vi "ReadAI.vi"(8 "error in (no error)":errorcluster, 11 "FPGA VI Reference In":refnum<k20>) -> (0 "error out":errorcluster, 2 "AI_readValues":dbl[](array[numeric]), 3 "FPGA VI Reference Out":refnum<k20>)   [LabVIEW 2020, in "FPGA_IO.lvlib"]
doc: "Read AI values from the FPGA\nChannels: C/AI0, C/AI1"
uses:
  FPGA_IO.lvlib
  <vilib>/Utility/error.llb/Error Cluster From Error Code.vi
  <vilib>/rvi/errors/niLvFpgaAdjustHostInterfaceError.vi
  <vilib>/rvi/interface/nirviReadWriteControl/nirviReadWriteControl.xnode
  NiFpgaLv.dll
  <vilib>/rvi/interface/Simulation/niFpgaSimulationCallBeginRW.vi
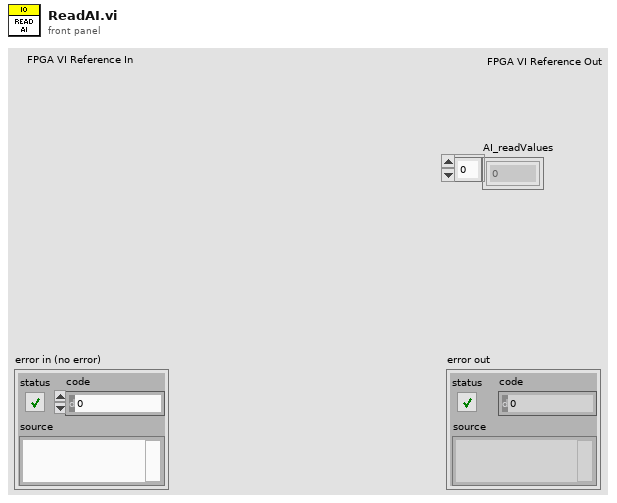
[diagram p1: front panel]
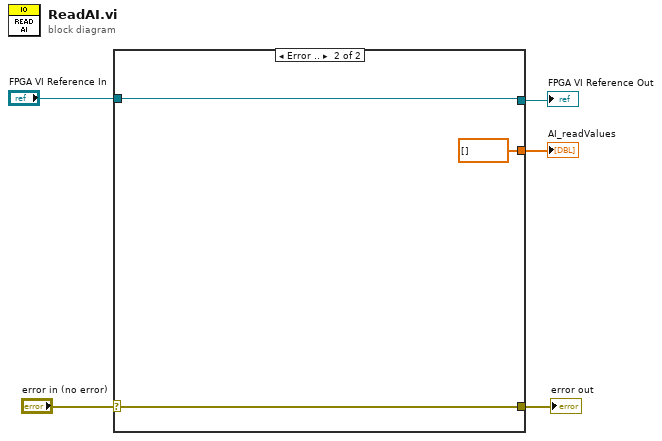
[diagram p0: block diagram]
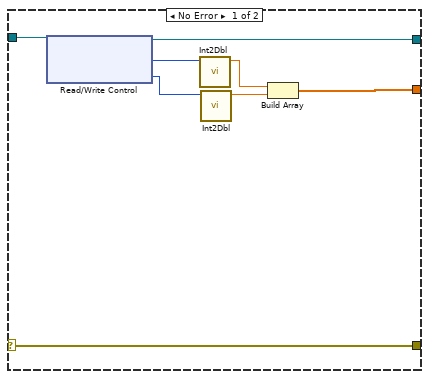
[diagram p2: hidden frame]
diagram:
  n1 = case shown="Error .." "error in (no error)" {
    selector: "error in (no error)" -> [w6 w14]
    tunnel: "FPGA VI Reference In" -> [w13 w15]
    tunnel: [w12 w15] -> w4
    tunnel: [w7 dbl[] []] -> w3
    tunnel: [w6 w14] -> w1
    frame No Error {
      n2 = xnode "Read/Write Control"("FPGA VI Reference In"=w13) -> ("FPGA VI Reference Out"=w12:refnum<k20>, "C_AI0_readValue"=w11:i16, "C_AI1_readValue"=w10:i16)  [unwired: 1 in, 1 out]
      n3 = call "Int2Dbl.vi"("AI_raw"=w11) -> ("AI_converted [V]"=w9:dbl)  [unwired: 10 in]
      n4 = call "Int2Dbl.vi"("AI_raw"=w10) -> ("AI_converted [V]"=w8:dbl)  [unwired: 10 in]
      n5 = Build Array(w9, w8) -> (w7:dbl[])
    }
    frame Error {
    }
  }
  "FPGA VI Reference Out" <- w4
  "AI_readValues" <- w3
  "error out" <- w1
